vi "errorHandler.vi"(6 "code":i32, 8 "error in":errorcluster) -> (0 "error out":errorcluster)   [LabVIEW 2020, in "camera.lvclass"]
uses:
  camera.lvclass
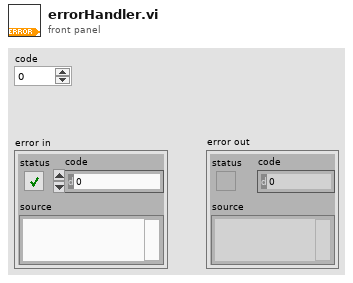
[diagram p1: front panel]
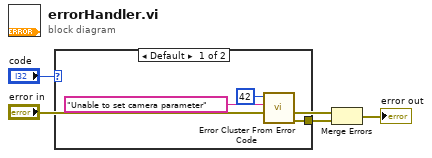
[diagram p0: block diagram]
diagram:
  n1 = case shown="Default" "code" {
    tunnel: [w7 _] -> w1
    frame Default {
      n2 = call <vilib>:"Error Cluster From Error Code.vi"("error message (\"\")"="Unable to set camera parameter" ("error message (\"\")"), "error code (0)"=42) -> ("error out"=w7:errorcluster)  [unwired: 7 in]
    }
    frame 1 {
    }
  }
  n3 = Merge Errors("error in", w1) -> (→"error out":errorcluster)
